vi "Load Cell Calculations.vi"(10 "Ball Offset":dbl, 11 "Load Cell Value":dbl) -> (3 "Multiplier":dbl)   [LabVIEW 2012]
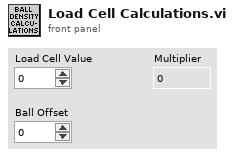
[diagram p1: front panel]
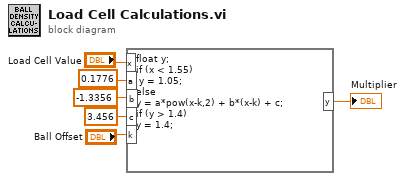
[diagram p0: block diagram]
diagram:
  n1 = formula code="float y;\nif (x < 1.55)\n y = 1.05;\nelse \ny = a*pow(x-k,2) + b*(x-k) + c;\nif (y > 1.4) \ny = 1.4;"("x"="Load Cell Value", "k"="Ball Offset", "a"=0.1776 ("input variable"), "b"=-1.3356 ("input variable"), "c"=3.456 ("input variable")) -> ("y"=→"Multiplier":dbl)
